vi "Main4Diposits.vi"() -> ()   [LabVIEW 2019]
panel:
  out "Boolean 4":bool
  in  "Dipòsit 4":dbl(slide) scale=0.0..10000.0
  out "OPERACIÓ NORMAL":bool
  out "ALARMA":bool
  in  "stop":bool
  out "Boolean 3":bool
  out "Boolean 2":bool
  out "Boolean":bool
  in  "Límit buit":dbl(slide) scale=0.0..10000.0
  in  "Dipòsit 3":dbl(slide) scale=0.0..10000.0
  in  "Dipòsit 2":dbl(slide) scale=0.0..10000.0
  in  "Dipòsit 1":dbl(slide) scale=0.0..10000.0
  # "DISSENY D'UN CIRCUIT LÒGIC PER A UNA PLANTA DEPURADORA"
  # "ESTAT PLANTA\nDEPURADORA"
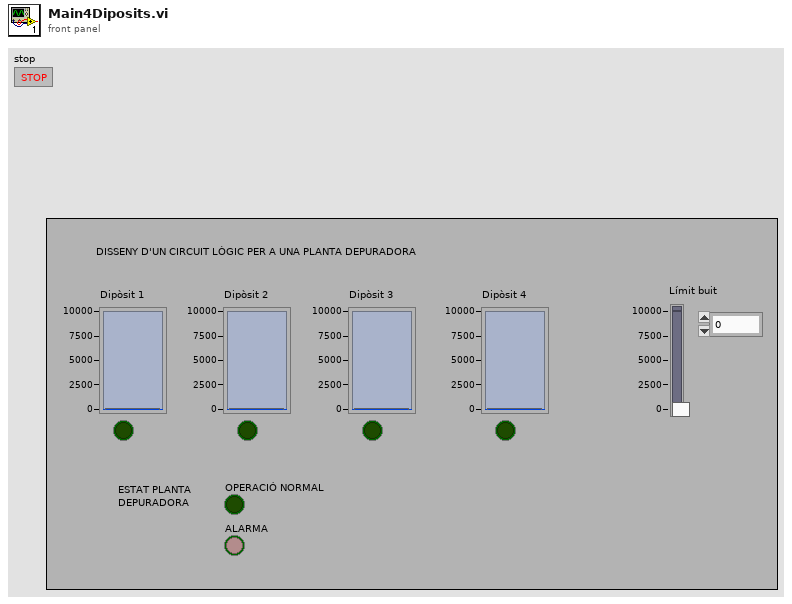
[diagram p1: front panel]
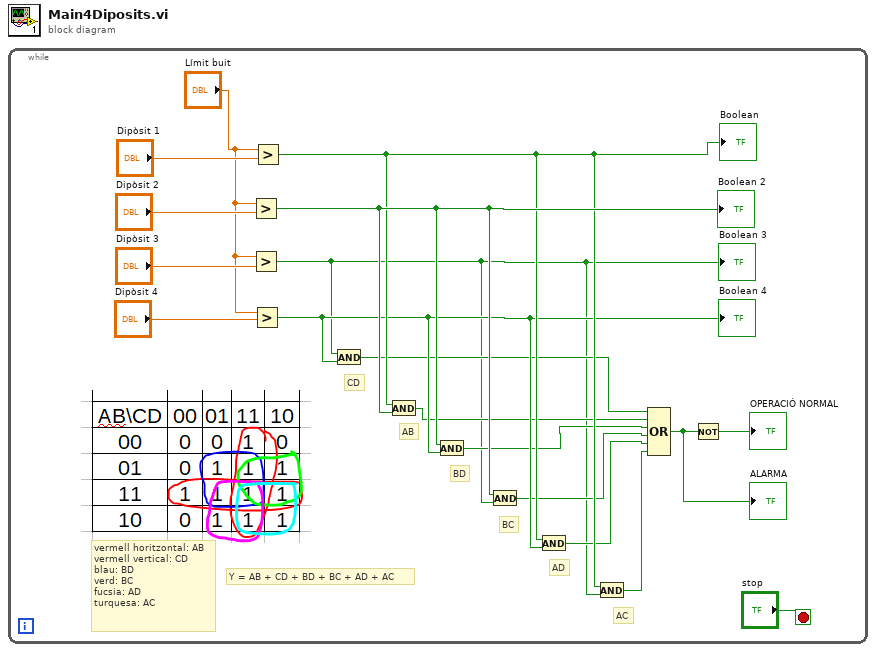
[diagram p0: block diagram]
diagram:
  n1 = while {
    stop <- "stop" stop-if-true
    # "Y = AB + CD + BD + BC + AD + AC"
    # "vermell horitzontal: AB\nvermell vertical: CD\nblau: BD\nverd: BC\nfucsia: AD\nturquesa: AC"
    # "AC"
    # "AD"
    # "BC"
    # "BD"
    # "AB"
    # "CD"
    n2 = Greater?(x="Límit buit", y="Dipòsit 2") -> (0:w12:bool)
    "Boolean 2" <- w12
    n3 = Greater?(x="Límit buit", y="Dipòsit 3") -> (0:w1:bool)
    "Boolean 3" <- w1
    n4 = Greater?(x="Límit buit", y="Dipòsit 4") -> (0:w10:bool)
    "Boolean 4" <- w10
    n5 = Greater?(x="Límit buit", y="Dipòsit 1") -> (0:w11:bool)
    "Boolean" <- w11
    n6 = And(x=w1, y=w10) -> (x .and. y?=w9:bool)
    n7 = And(x=w11, y=w12) -> (x .and. y?=w8:bool)
    n8 = And(x=w12, y=w10) -> (x .and. y?=w7:bool)
    n9 = And(x=w12, y=w1) -> (x .and. y?=w6:bool)
    n10 = And(x=w11, y=w10) -> (x .and. y?=w5:bool)
    n11 = And(x=w11, y=w1) -> (x .and. y?=w4:bool)
    n12 = Compound Arithmetic op=OR(w9, w8, w7, w6, w5, w4) -> (w2:bool)
    "ALARMA" <- w2
    n13 = Not(x=w2) -> (.not. x?=→"OPERACIÓ NORMAL":bool)
  }
